vi "Get Time.vi"(11 "error in (no error)":errorcluster) -> (2 "Time (ns)":i64, 3 "error out":errorcluster)   [LabVIEW 2021, in "CIFCorePlugin.lvclass"]
uses:
  CIFCorePlugin.lvclass
  <vilib>/CIF Foundation/CIF Utilities/Time/System Time/LabVIEW Time to TAI Time.vi
  CIFCorePlugin.lvclass/CIFCorePlugin.ctl
  <vilib>/CIF Foundation/CIF Utilities/Time/Time_CIF_U.lvlib
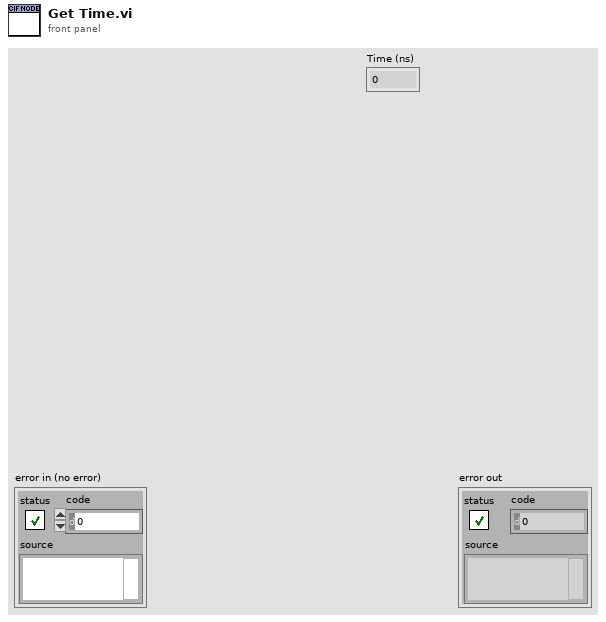
[diagram p1: front panel]
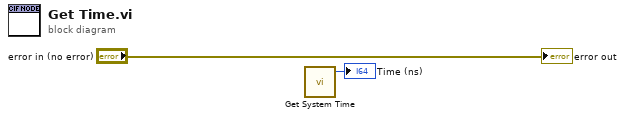
[diagram p0: block diagram]
diagram:
  n1 = call <vilib>:"Get System Time.vi"() -> ("Time (ns)"=→"Time (ns)":i64)  [unwired: 5 in]
  "error out" <- "error in (no error)"
